vi "Acquire.vi"(8 "error in (no error)":errorcluster, 11 "Hardware Resources in":T1) -> (0 "error out":errorcluster, 2 "data":waveform(dbl)[](array[waveform]), 3 "Hardware Resources out":T1)   [LabVIEW 2021]
doc: "Perform the acquisition. Replace the contents of this diagram with calls to acquisition hardware."
uses:
  <resource>/objmgr/daqmx.rc
  <vilib>/DAQmx/read.llb/DAQmx Read (Analog 1D Wfm NChan NSamp).vi
  Hardware Configuration.ctl
  Acquisition/Task Cluster.ctl
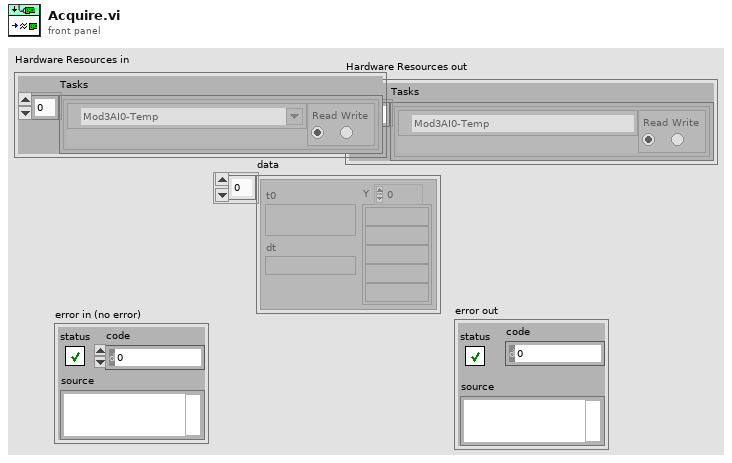
[diagram p1: front panel]
types:
  T1 = typedef "DAQ Write.lvlib/Hardware Configuration.ctl" = cluster{"Tasks":T2[]}
  T2 = typedef "Task Cluster.ctl" = cluster{"DAQmx Task":refnum<k21>, "Read-Write Radio":enum32{"Read", "Write"}}
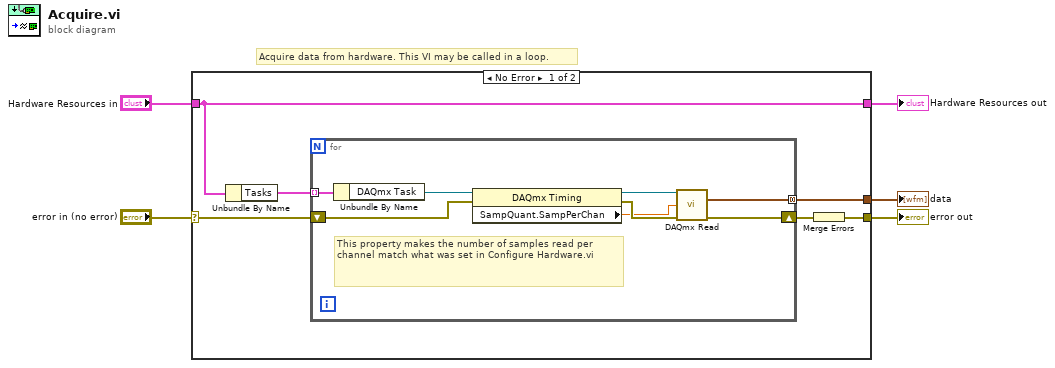
[diagram p0: block diagram]
diagram:
  # "Acquire data from hardware. This VI may be called in a loop."
  n1 = case shown="No Error" "error in (no error)" {
    selector: "error in (no error)" -> [w7 w20]
    tunnel: [w11 w20] -> w4
    tunnel: "Hardware Resources in" -> [w10 w21]
    tunnel: [w10 w21] -> w2
    tunnel: [w6 _] -> w1
    frame No Error {
      n2 = Unbundle By Name(w10) -> ("Tasks"=w8:T2[])
      n3 = for {
        tunnel: [w12] -> w6 mode=concatenating
        tunnel: w8 -> [w18] mode=indexing
        shift-right: [w19] -> w9
        shift-left: w7 -> [w16]
        # "This property makes the number of samples read per channel match what was set in Configure Hardware.vi"
        n4 = Unbundle By Name(w18) -> ("DAQmx Task"=w13:refnum<k21>)
        n5 = property class="DAQmx Timing"(reference=w13, error in=w16) -> (reference out=w17:refnum<k21>, error out=w15:errorcluster, "SampQuant.SampPerChan"=w14:dbl)
        n6 = call-poly <vilib>:"DAQmx Read.vi"("task/channels in"=w17, "number of samples per channel"=w14, "error in"=w15) -> ("data"=w12:waveform(dbl)[], "error out"=w19:errorcluster)  [unwired: 10 in, 1 out]
      }
      n7 = Merge Errors(w9) -> (w11:errorcluster)
    }
    frame Error {
    }
  }
  "Hardware Resources out" <- w2
  "error out" <- w4
  "data" <- w1
